vi "myRIO v1.2 Open AI.vi"(7 "Allow multiple opens?":bool, 8 "error in (no error)":errorcluster, 10 "Channel Names":string[](array[string]), 11 "Resource name":T5 caption="RIO Device") -> (0 "error out":errorcluster, 1 "AI Scale Constants List":T1, 2 "AI Channel List":T6, 3 "myRIO Ref Out":T3)   [LabVIEW 2021]
uses:
  <vilib>/myRIO/Common/Instrument Driver Framework/myRIO v1.0/AI/typedefs/AI Channels List.ctl
  <vilib>/myRIO/Common/Instrument Driver Framework/myRIO v1.0/AI/typedefs/AI Channels Enum.ctl
  <vilib>/userDefined/High Color/nirio_resource_hc.ctl
  <vilib>/myRIO/Common/Instrument Driver Framework/Utilities/typedefs/myRIO v1.0 Reference.ctl
  <vilib>/myRIO/Common/Instrument Driver Framework/Utilities/typedefs/Generic FPGA Reference.ctl
  <vilib>/myRIO/Common/Instrument Driver Framework/Utilities/typedefs/Analog Scaling Constants List.ctl
  <vilib>/myRIO/Common/Instrument Driver Framework/Utilities/typedefs/Analog Scaling Constants.ctl
  <vilib>/myRIO/Common/Instrument Driver Framework/myRIO v1.0/AI/typedefs/myRIO v1.2 AI Channels Enum.ctl
  <vilib>/myRIO/Common/Instrument Driver Framework/myRIO v1.0/AI/vis/myRIO v1.0 Build MUX Configuration AI.vi
  <vilib>/myRIO/Common/Instrument Driver Framework/myRIO v1.0/Resource Manager/vis/myRIO v1.0 Reserve Channel List.vi
  <vilib>/myRIO/Common/Instrument Driver Framework/myRIO v1.0/Resource Manager/vis/myRIO v1.0 Reserve Channel.vi
  <vilib>/myRIO/Common/Instrument Driver Framework/myRIO v1.0/Resource Manager/vis/myRIO v1.0 Unreserve Channel.vi
  <vilib>/myRIO/Common/Instrument Driver Framework/myRIO v1.0/Resource Manager/vis/myRIO v1.0 Build Mutex Name.vi
  <vilib>/Utility/VariantDataType/GetNumericInfo.vi
  <vilib>/Utility/error.llb/Error Cluster From Error Code.vi
  <vilib>/myRIO/Common/Instrument Driver Framework/Utilities/vis/IO Manager.vi
  <vilib>/myRIO/Common/Instrument Driver Framework/Utilities/vis/Configuration Manager.vi
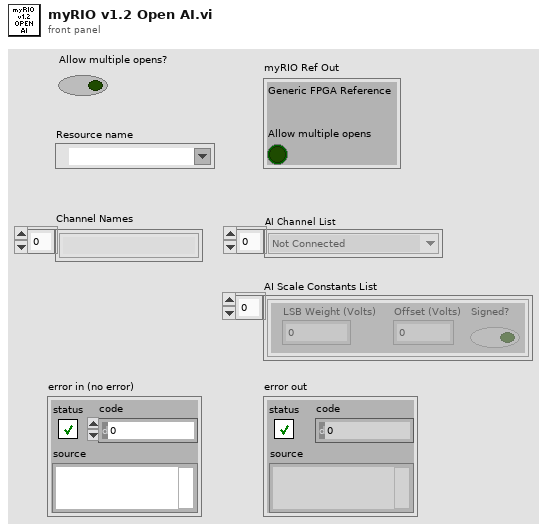
[diagram p1: front panel]
types:
  T1 = typedef "Analog Scaling Constants List.ctl" = T2[]
  T2 = typedef "Analog Scaling Constants.ctl" = cluster{"LSB Weight (Volts)":dbl, "Offset (Volts)":dbl, "Signed?":bool}
  T3 = typedef "myRIO v1.0 Reference.ctl" = cluster{"Generic FPGA Reference":T4, "Allow multiple opens":bool}
  T4 = typedef "Generic FPGA Reference.ctl" = refnum<k20>
  T5 = typedef "nirio_resource_hc.ctl" = tag
  T6 = typedef "AI Channels List.ctl" = T7[]
  T7 = typedef "AI Channels Enum.ctl" = enum16{"Not Connected", "AudioIn/Left", "AudioIn/Right", "C/AI0", "C/AI1", "A/AI0", "A/AI1", "A/AI2", "A/AI3", "A/AI4", "A/AI5", "A/AI6", "A/AI7", "B/AI0", "B/AI1", "B/AI2", "B/AI3", "B/AI4", "B/AI5", "B/AI6", "B/AI7", "AI/AI0", "AI/AI1", "AI/AI2", "AI/AI3", "A/AI0 (DIFF)", "A/AI1 (DIFF)", "A/AI2 (DIFF)", "A/AI3 (DIFF)", "B/AI0 (DIFF)", "B/AI1 (DIFF)", "B/AI2 (DIFF)", "B/AI3 (DIFF)"}
  T8 = typedef "myRIO v1.2 AI Channels Enum.ctl" = enum16{"Not Connected", "A/AI0", "A/AI1", "A/AI2", "A/AI3", "B/AI0", "B/AI1", "B/AI2", "B/AI3"}
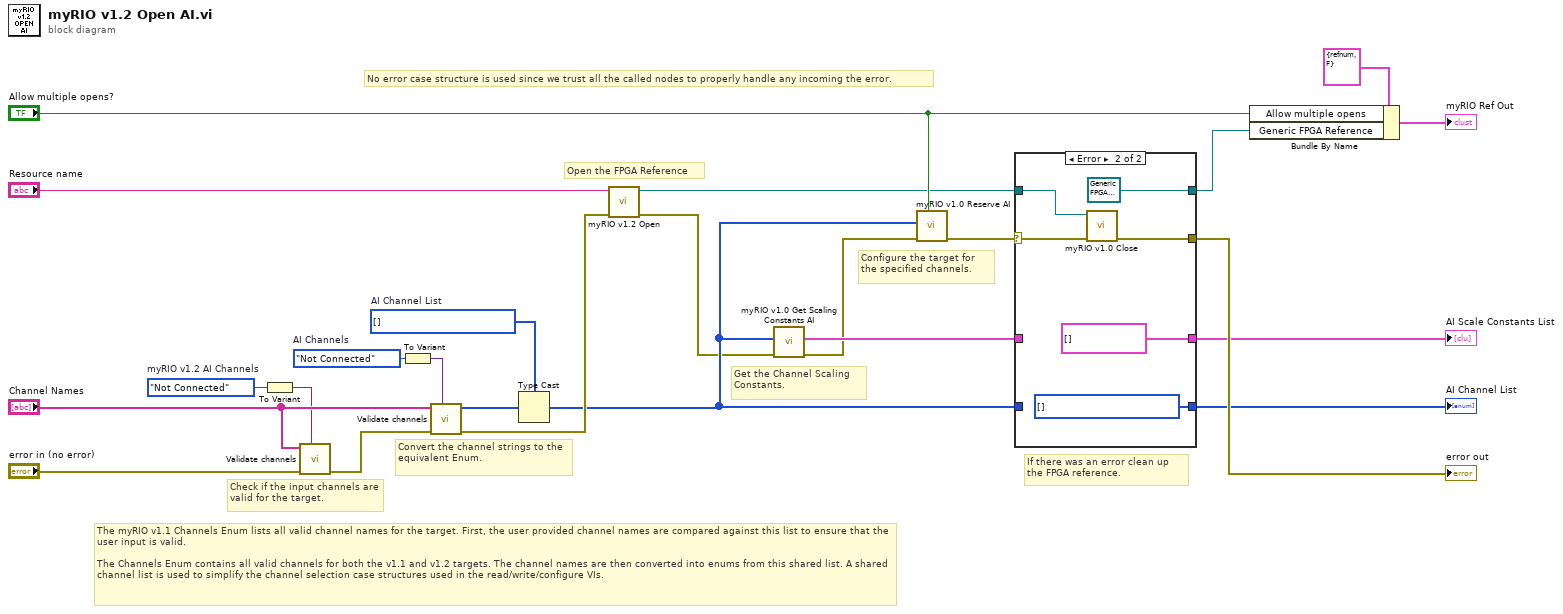
[diagram p0: block diagram]
diagram:
  w4 = AI_Channels_Enum."Not Connected"  # AI Channels
  w2 = myRIO_v1.2_AI_Channels_Enum."Not Connected"  # myRIO v1.2 AI Channels
  w18 = T6 [] items=["Not Connected", "AudioIn/Left", "AudioIn/Right", "C/AI0", "C/AI1", "A/AI0", "A/AI1", "A/AI2", "A/AI3", "A/AI4", "A/AI5", "A/AI6", "A/AI7", "B/AI0", "B/AI1", "B/AI2", "B/AI3", "B/AI4", "B/AI5", "B/AI6", "B/AI7", "AI/AI0", "AI/AI1", "AI/AI2", "AI/AI3", "A/AI0 (DIFF)", "A/AI1 (DIFF)", "A/AI2 (DIFF)", "A/AI3 (DIFF)", "B/AI0 (DIFF)", "B/AI1 (DIFF)", "B/AI2 (DIFF)", "B/AI3 (DIFF)"]  # AI Channel List
  # "Get the Channel Scaling Constants."
  # "The myRIO v1.1 Channels Enum lists all valid channel names for the target. First, the user provided channel names are compared against this list to ensure that the user input is valid.\n\nThe Channels Enum contains all valid channels for both the v1.1 and v1.2 targets. The channel names are then converted into enums from this shared list. A shared channel list is used to simplify the channel selection case structures used in the read/write/configure VIs."
  # "If there was an error clean up the FPGA reference."
  # "Configure the target for the specified channels."
  # "Open the FPGA Reference"
  # "No error case structure is used since we trust all the called nodes to properly handle any incoming the error."
  # "Convert the channel strings to the equivalent Enum."
  # "Check if the input channels are valid for the target."
  n1 = To Variant(anything=w2) -> (Variant=w1:variant)
  n2 = call <vilib>:"Validate channels.vi"("Channels Enum Variant"=w1, "error in (no error)"="error in (no error)", "Channel Names"="Channel Names") -> ("error out"=w23:errorcluster)  [unwired: 7 in, 1 out]
  n3 = To Variant(anything=w4) -> (Variant=w3:variant)
  n4 = call <vilib>:"Validate channels.vi"("Channels Enum Variant"=w3, "error in (no error)"=w23, "Channel Names"="Channel Names") -> ("error out"=w19:errorcluster, "Index Array"=w17:u16[])  [unwired: 7 in]
  n5 = Type Cast(type=w18, x=w17) -> (*(type *) &x=w11:T6)
  n6 = call <vilib>:"myRIO v1.2 Open.vi"("error in (no error)"=w19, "Resource name"="Resource name") -> ("error out"=w6:errorcluster, "myRIO FPGA Ref Out"=w10:T4)  [unwired: 8 in]
  n7 = call <vilib>:"myRIO v1.0 Get Scaling Constants AI.vi"("error in (no error)"=w6, "Channel List"=w11) -> ("error out"=w5:errorcluster, "Scale Constants Array"=w9:T1)  [unwired: 8 in]
  n8 = call <vilib>:"myRIO v1.0 Reserve AI.vi"("Allow multiple opens?"="Allow multiple opens?", "error in (no error)"=w5, "AI Channel List"=w11) -> ("error out"=w7:errorcluster)  [unwired: 8 in]
  n9 = case shown="Error" w7 {
    selector: w7 -> [w28 w34]
    tunnel: [w25 T4 refnum ("myRIO FPGA Ref Out")] -> w14
    tunnel: [w28 w33] -> w21
    tunnel: [w27 w31] -> w16
    tunnel: w11 -> [w27 _]
    tunnel: w10 -> [w25 w30]
    tunnel: w9 -> [w26 _]
    tunnel: [w26 T1 [] ("Scale Constants Array")] -> w8
    frame No Error {
    }
    frame Error {
      w31 = T6 [] items=["Not Connected", "AudioIn/Left", "AudioIn/Right", "C/AI0", "C/AI1", "A/AI0", "A/AI1", "A/AI2", "A/AI3", "A/AI4", "A/AI5", "A/AI6", "A/AI7", "B/AI0", "B/AI1", "B/AI2", "B/AI3", "B/AI4", "B/AI5", "B/AI6", "B/AI7", "AI/AI0", "AI/AI1", "AI/AI2", "AI/AI3", "A/AI0 (DIFF)", "A/AI1 (DIFF)", "A/AI2 (DIFF)", "A/AI3 (DIFF)", "B/AI0 (DIFF)", "B/AI1 (DIFF)", "B/AI2 (DIFF)", "B/AI3 (DIFF)"]
      n10 = call <vilib>:"myRIO v1.0 Close.vi"("error in (no error)"=w34, "myRIO FPGA Ref In"=w30) -> ("error out"=w33:errorcluster)  [unwired: 9 in]
    }
  }
  "AI Channel List" <- w16
  "error out" <- w21
  "AI Scale Constants List" <- w8
  n11 = Bundle By Name(cluster=T3 {"Generic FPGA Reference"=refnum, "Allow multiple opens"=FALSE} ("myRIO Hardware Reference"), "Allow multiple opens"="Allow multiple opens?", "Generic FPGA Reference"=w14) -> (→"myRIO Ref Out":T3)
